vi "U8-U32.vi"(1 "数组":u8[](array[numeric]), 3 "error in (no error)":errorcluster caption="错误输入（无错误）") -> (8 "32位整型":i32, 10 "error out":errorcluster caption="错误输出")   [LabVIEW 2014]
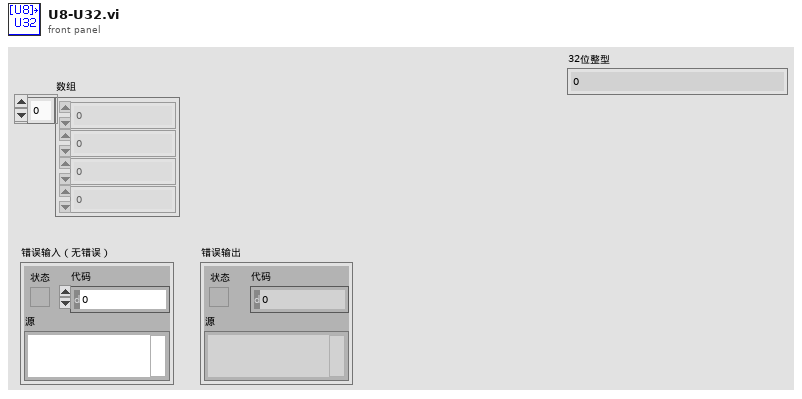
[diagram p1: front panel]
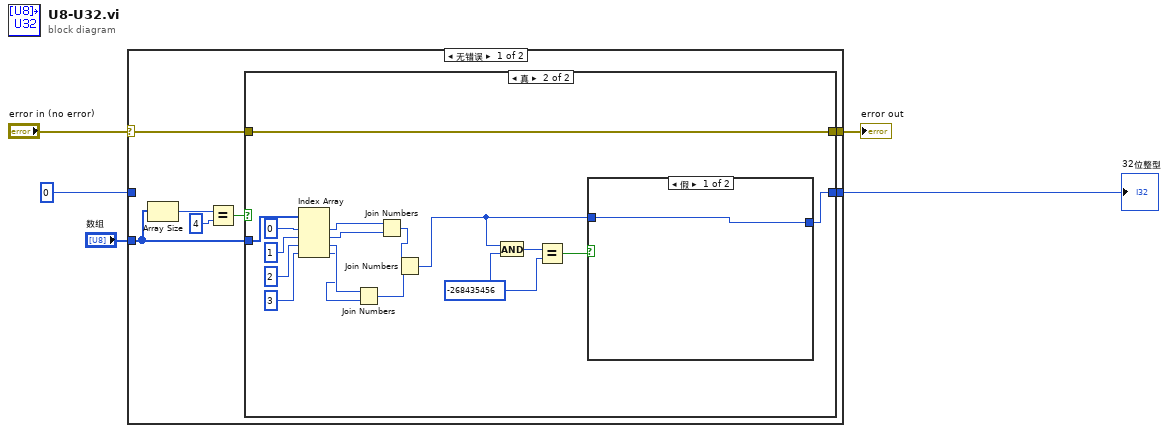
[diagram p0: block diagram]
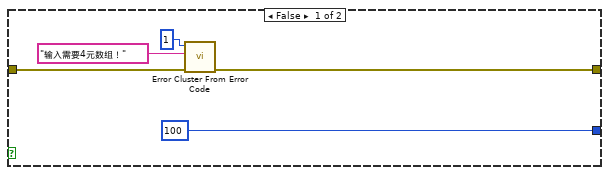
[diagram p2: hidden frame]
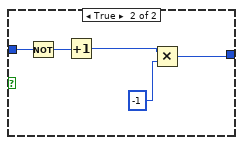
[diagram p3: hidden frame]
diagram:
  n1 = case shown="无错误" "error in (no error)" {
    selector: "error in (no error)" -> [w12 w42]
    tunnel: [w11 w42] -> w4
    tunnel: "数组" -> [w7 _]
    tunnel: 0 -> [_ w41]
    tunnel: [w6 w41] -> w1
    frame No Error {
      n2 = Array Size(array=w7) -> (size(s)=w10:i32)
      n3 = Equal?(x=w10, y=4) -> (x = y?=w8:bool)
      n4 = case shown="真" w8 {
        tunnel: w12 -> [w15 w30]
        tunnel: [w14 w30] -> w11
        tunnel: w7 -> [_ w31]
        tunnel: [100 w18] -> w6
        frame False {
          n5 = call <vilib>:"Error Cluster From Error Code.vi"("error in (no error)"=w15, "error message (\"\")"="输入需要4元数组！" ("error message (\"\")"), "error code (0)"=1) -> ("error out"=w14:errorcluster)  [unwired: 6 in]
        }
        frame True {
          w27 = -268435456 ("y")
          n6 = Index Array(array=w31, index #1=0 ("索引"), index #2=1 ("索引"), index #3=2 ("索引"), index #4=3 ("索引")) -> (element #1=w22:u8, element #2=w21:u8, element #3=w20:u8, element #4=w19:u8)
          n7 = Join Numbers(hi=w20, lo=w19) -> ((hi.lo)=w24:u16)
          n8 = Join Numbers(hi=w22, lo=w21) -> ((hi.lo)=w25:u16)
          n9 = Join Numbers(hi=w25, lo=w24) -> ((hi.lo)=w23:u32)
          n10 = And(x=w23, y=w27) -> (x .and. y?=w28:u32)
          n11 = Equal?(x=w28, y=w27) -> (x = y?=w26:bool)
          n12 = case shown="假" w26 {
            tunnel: w23 -> [w35 w39]
            tunnel: [w35 w37] -> w18
            frame False {
            }
            frame True {
              n13 = Not(x=w39) -> (.not. x?=w40:u32)
              n14 = Increment(x=w40) -> (x+1=w36:u32)
              n15 = Multiply(x=w36, y=-1) -> (x*y=w37:u32)
            }
          }
        }
      }
    }
    frame Error {
    }
  }
  "error out" <- w4
  "32位整型" <- w1
